vi "Method_Const.vi"(4 "Value":ext, 5 "Input A":T1) -> (1 "Result":T1)   [LabVIEW 2021, in "Divide_EXT.lvclass"]
uses:
  Divide_EXT.lvclass
  Abs Type.ctl
  Abs_Types/Extended Float/Abs_Extended Float.lvclass
  C:/Program Files (x86)/National Instruments/LabVIEW 2021/vi.lib/TSA/Abstract Data Classes/Abs_Types/Numeric/Abs_Numeric.lvclass
  C:/TSA/LV_Abstract/Source/Functions/Support/Function/Two Terminal/EXT/AbsFunc_Two Term_EXT.lvclass
  C:/Program Files (x86)/National Instruments/LabVIEW 2021/vi.lib/TSA/Abstract Data Classes/Abs_Types/Extended Float/Abs_Extended Float.lvclass
  Support/Function/Two Terminal/EXT/AbsFunc_Two Term_EXT.lvclass/AbsFunc_Two Term_EXT.ctl
  Support/Function/Two Terminal/EXT/Properties/Write Numeric A.vi
  Support/Function/Two Terminal/EXT/Properties/Write Numeric B.vi
  Constants/Support/EXT/Const_EXT.lvclass
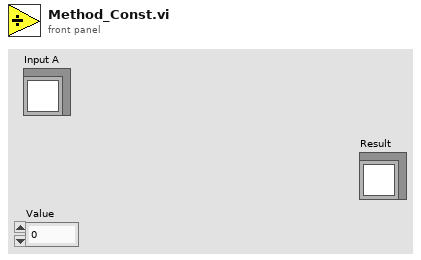
[diagram p1: front panel]
types:
  T1 = typedef "Divide_EXT.lvclass/Abs Type.ctl" = refnum<class "Abs_Extended Float.lvclass">
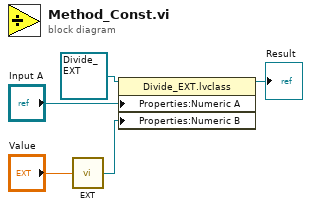
[diagram p0: block diagram]
diagram:
  n1 = call "EXT.vi"("Value"="Value") -> ("Constant"=w2:refnum<class "Abs_Extended Float.lvclass">)  [unwired: 4 in]
  n2 = property class="Divide_EXT.lvclass"(reference=refnum<class "Divide_EXT.lvclass"> refnum ("Functions.lvlib:Numeric.lvlib:Divide.lvclass"), "Properties:Numeric A"="Input A", "Properties:Numeric B"=w2) -> (reference out=→"Result":refnum<class "Divide_EXT.lvclass">)  [unwired: 1 in, 1 out]
